vi "Load Vantage Calibration V.vi"(8 "error in (no error)":errorcluster, 11 "vantageCalibration":T1) -> (0 "error out":errorcluster, 2 "function return":i32, 3 "vantageCalibration out":T1)   [LabVIEW 2009, in "VantagePro.lvlib"]
doc: "DllAccess int _stdcall LoadVantageCalibration_V(CurrentVantageCalibration &vantageCalibration);"
uses:
  VantagePro.lvlib
  <userlib>/VantagePro/VantagePro.dll
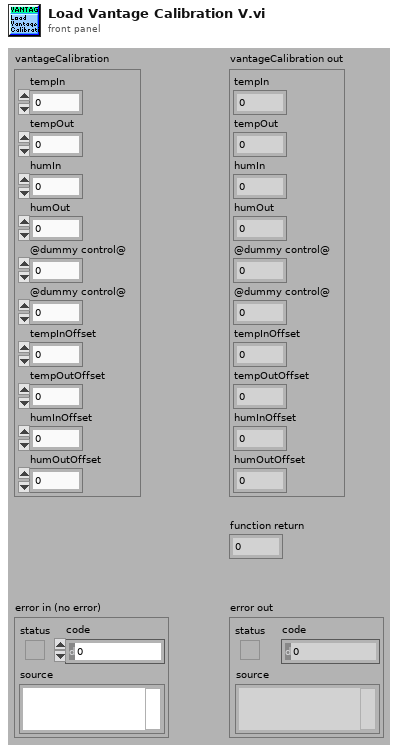
[diagram p1: front panel]
types:
  T1 = cluster{"tempIn":sgl, "tempOut":sgl, "humIn":u8, "humOut":u8, "@dummy control@":i8, "@dummy control@":i8, "tempInOffset":sgl, "tempOutOffset":sgl, "humInOffset":i8, "humOutOffset":i8}
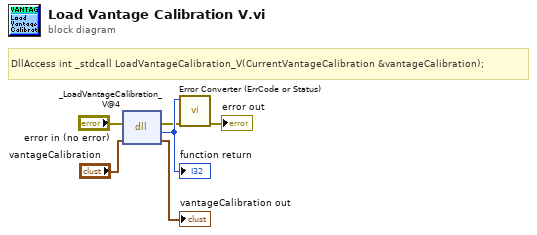
[diagram p0: block diagram]
diagram:
  # "DllAccess int _stdcall LoadVantageCalibration_V(CurrentVantageCalibration &vantageCalibration);"
  n1 = dll-call lib="C:/Program Files/National Instruments/LabVIEW 2010/user.lib/VantagePro/VantagePro.*" fn="_LoadVantageCalibration_V@4"(error in="error in (no error)", "vantageCalibration"="vantageCalibration") -> (error out=w2:errorcluster, w6:i32, "vantageCalibration"=→"vantageCalibration out":T1)  [unwired: 2 in, 1 out]
  "function return" <- w6
  n2 = call "Error Converter (ErrCode or Status).vi"("error in (no error)"=w2, "error code"=w6) -> ("error out"=→"error out":errorcluster)  [unwired: 9 in]
